vi "Throw Event.vi"(8 "error in (no error)":errorcluster, 9 "Event":T1=enum."Closed", 10 "Panel":string, 11 "Panel Registry in":refnum<class "Panel Registry.lvclass">) -> (0 "error out":errorcluster, 3 "Panel Registry out":refnum<class "Panel Registry.lvclass">)   [LabVIEW 2020, in "Panel.lvlib" / "Panel Registry.lvclass"]
doc: "Throws an event in the Panel Registry.\n\n----\nPlease see the following web address for additional documentation and tutorial information:\nhttp://www.mooregoodideas.com/mgi-panel-manager/\n\nAuthor: Derek Trepanier\n\nCopyright (c) 2018, Moore Good Ideas, Inc.\n\nAll rights reserved.\n\nRedistribution and use in source and binary forms, with or without modification, are permitted provided that the following conditions are met:\n\n * Redistributions of source code must retain the above copyright notice, this list of conditions and the following disclaimer.\n * Redistributions in binary form must reproduce the above copyright notice, this list of conditions and the following disclaimer in the documentation and/or other materials provided with the distribution.\n * Neither the name of Moore Good Ideas, Inc. nor the names of its contributors may be used to endorse or promote products derived from this software without specific prior written permission.\n\nTHIS SOFTWARE IS PROVIDED BY THE COPYRIGHT HOLDERS AND CONTRIBUTORS \"AS IS\" AND ANY EXPRESS OR IMPLIED WARRANTIES, INCLUDING, BUT NOT LIMITED TO, THE IMPLIED WARRANTIES OF MERCHANTABILITY AND FITNESS FOR A PARTICULAR PURPOSE ARE DISCLAIMED. IN NO EVENT SHALL THE COPYRIGHT OWNER OR CONTRIBUTORS BE LIABLE FOR ANY DIRECT, INDIRECT, INCIDENTAL, SPECIAL, EXEMPLARY, OR CONSEQUENTIAL DAMAGES (INCLUDING, BUT NOT LIMITED TO, PROCUREMENT OF SUBSTITUTE GOODS OR SERVICES; LOSS OF USE, DATA, OR PROFITS; OR BUSINESS INTERRUPTION) HOWEVER CAUSED AND ON ANY THEORY OF LIABILITY, WHETHER IN CONTRACT, STRICT LIABILITY, OR TORT (INCLUDING NEGLIGENCE OR OTHERWISE) ARISING IN ANY WAY OUT OF THE USE OF THIS SOFTWARE, EVEN IF ADVISED OF THE POSSIBILITY OF SUCH DAMAGE."
uses:
  <vilib>/MGI/Panel Manager/Panel/Panel Registry/Panel Registry.lvclass
  <vilib>/MGI/Panel Manager/Panel/Panel Helper/Events.ctl
  <vilib>/MGI/Panel Manager/Panel/Panel Registry/Panel Registry.lvclass/Panel Registry.ctl
  <vilib>/MGI/Panel Manager/Panel/Panel Helper/Panel Events.ctl
  <vilib>/MGI/Panel Manager/Panel/Panel Helper/Panel Helper.lvclass
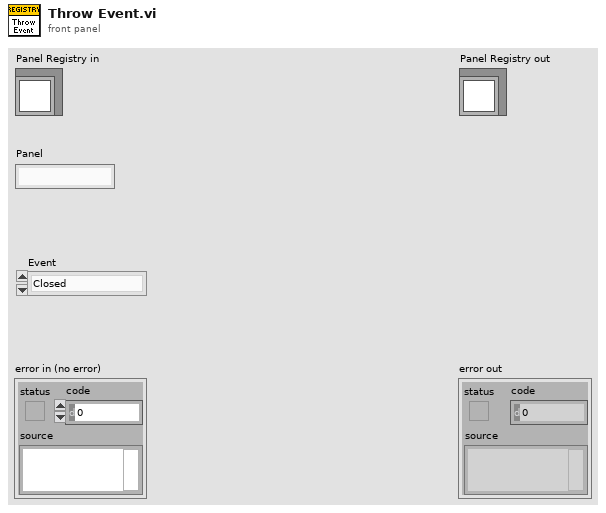
[diagram p1: front panel]
types:
  T1 = typedef "Panel.lvlib/Panel Helper.lvclass/Events.ctl" = enum16{"Initialized", "Shown", "Hidden", "Closed"}
  T2 = typedef "Panel.lvlib/Panel Helper.lvclass/Panel Events.ctl" = cluster{"My Panel":refnum<user-event>, "Top Level Initialized":refnum<user-event>}
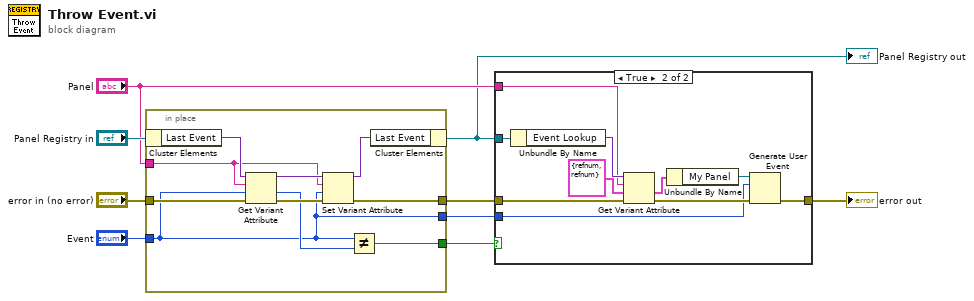
[diagram p0: block diagram]
diagram:
  n1 = in-place {
    in-place-border: "Panel" -> [w17]
    in-place-border: "Event" -> [w10]
    in-place-border: [w15] -> w6
    in-place-border: "error in (no error)" -> [w13]
    in-place-border: [w11] -> w3
    in-place-border: [w10] -> w1
    n2 = in-place-cluster #1("Panel Registry in") -> ("Last Event"=w19:variant)
    n3 = Get Variant Attribute(Variant=w19, name=w17, default value (empty Variant)=w10, error in=w13) -> (duplicate Variant=w18:variant, value=w12:T1, error out=w14:errorcluster)  [unwired: 1 out]
    n4 = Set Variant Attribute(Variant=w18, name=w17, value=w10, error in=w14) -> (Variant out=w16:variant, error out=w15:errorcluster)  [unwired: 1 out]
    n5 = Not Equal?(x=w10, y=w12) -> (x != y?=w11:bool)
    n6 = in-place-cluster #1("Last Event"=w16) -> (w2:refnum<class "Panel Registry.lvclass">)
  }
  "Panel Registry out" <- w2
  n7 = case shown="True" w3 {
    tunnel: w2 -> [_ w30]
    tunnel: "Panel" -> [_ w27]
    tunnel: w6 -> [w20 w23]
    tunnel: [w20 w22] -> w4
    tunnel: w1 -> [_ w21]
    frame False {
    }
    frame True {
      n8 = Unbundle By Name(w30) -> ("Event Lookup"=w29:variant)
      n9 = Get Variant Attribute(Variant=w29, name=w27, default value (empty Variant)=T2 {"My Panel"=refnum, "Top Level Initialized"=refnum} ("Events"), error in=w23) -> (value=w26:T2, error out=w24:errorcluster)  [unwired: 2 out]
      n10 = Unbundle By Name(w26) -> ("My Panel"=w25:refnum<user-event>)
      n11 = Generate User Event(user event=w25, event data cluster=w21, error in=w24) -> (error out=w22:errorcluster)  [unwired: 1 in, 1 out]
    }
  }
  "error out" <- w4
